vi "BRig_Host_prepareStoreLocation.vi"(8 "input_error":errorcluster, 10 "input_expPrefix":string) -> (0 "output_error":errorcluster, 2 "output_folderPath":string)   [LabVIEW 2014]
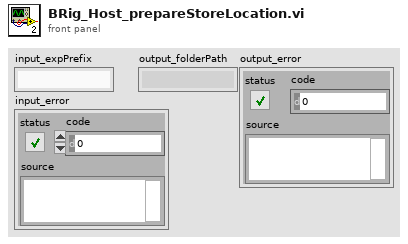
[diagram p1: front panel]
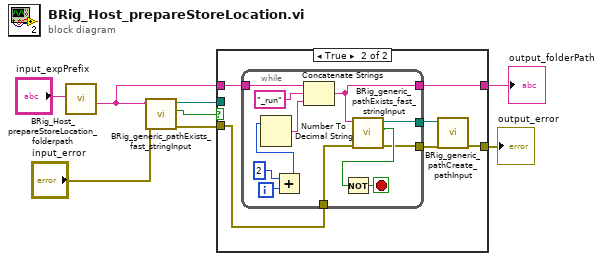
[diagram p0: block diagram]
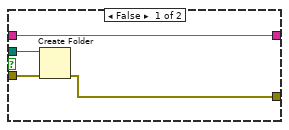
[diagram p2: hidden frame]
diagram:
  n1 = call "BRig_Host_prepareStoreLocation_folderpath.vi"("input_expPrefix"="input_expPrefix") -> ("output_folderPath"=w3:string)  [unwired: 10 in]
  n2 = call "BRig_generic_pathExists_fast_stringInput.vi"("input_error"="input_error", "input_filePath"=w3) -> ("output_error"=w6:errorcluster, "output_Iexist"=w5:bool, "output_filePath"=w4:path)  [unwired: 7 in]
  n3 = case shown="True" w5 {
    tunnel: w4 -> [w12 _]
    tunnel: w6 -> [w11 w16]
    tunnel: w3 -> [w10 w18]
    tunnel: [w10 w17] -> w7
    tunnel: [w9 w13] -> w2
    frame False {
      n4 = Create Folder(path (use dialog)=w12, error in=w11) -> (error out=w9:errorcluster)  [unwired: 1 in, 2 out]
    }
    frame True {
      n5 = while {
        tunnel: w18 -> [w30]
        tunnel: [w23] -> w17
        tunnel: [w22] -> w14
        tunnel: [w20] -> w15
        tunnel: w16 -> [w19]
        i -> [w27]
        stop <- w24 stop-if-true
        n6 = Add(x=2, y=w27) -> (x+y=w26:i32)
        n7 = Number To Decimal String(number=w26) -> (decimal integer string=w28:string)  [unwired: 1 in]
        n8 = Concatenate Strings(w30, "_run" ("string"), w28) -> (w23:string)
        n9 = call "BRig_generic_pathExists_fast_stringInput.vi"("input_error"=w19, "input_filePath"=w23) -> ("output_error"=w20:errorcluster, "output_Iexist"=w21:bool, "output_filePath"=w22:path)  [unwired: 7 in]
        n10 = Not(x=w21) -> (.not. x?=w24:bool)
      }
      n11 = call "BRig_generic_pathCreate_pathInput.vi"("input_error"=w15, "input_filePath"=w14) -> ("output_error"=w13:errorcluster)  [unwired: 8 in, 1 out]
    }
  }
  "output_folderPath" <- w7
  "output_error" <- w2
